vi "Create user events.vi"(8 "error in (no error)":errorcluster) -> (0 "error out":errorcluster, 3 "User events":T1)   [LabVIEW 2020, in "NI DAQ.lvlib"]
uses:
  NI DAQ.lvlib
  Task list.ctl
  Continuous aquisition params.ctl
  Controls/Acuisition type --typedef.ctl
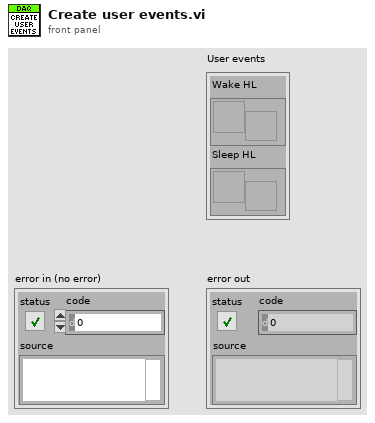
[diagram p1: front panel]
types:
  T1 = cluster{"Wake HL":refnum<user-event>, "Sleep HL":refnum<user-event>}
  T2 = typedef "NI DAQ.lvlib/Continuous aquisition params.ctl" = cluster{"Module ID":i32, "Task list":T3, "Timeout":i32, "Data in":variant, "DAQmx Task":refnum<k21>, "N samples":i32, "Acq type":T4}
  T3 = typedef "NI DAQ.lvlib/Task list.ctl" = enum16{"All", "DO task", "DI task", "AO task", "AI task", "CI task", "CO task", "TC task"}
  T4 = typedef "NI DAQ.lvlib/Acuisition type --typedef.ctl" = enum16{"Single", "Average", "Multiple"}
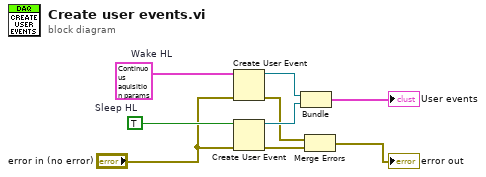
[diagram p0: block diagram]
diagram:
  w6 = TRUE  # Sleep HL
  w5 = T2 {"Module ID"=0, "Task list"=enum."All", "Timeout"=0, "Data in"=variant, "DAQmx Task"="", "N samples"=0, "Acq type"=enum."Single"}  # Wake HL
  n1 = Create User Event(user event datatype=w5, error in="error in (no error)") -> (user event=w7:refnum<user-event>, error out=w3:errorcluster)
  n2 = Create User Event(user event datatype=w6, error in="error in (no error)") -> (user event=w8:refnum<user-event>, error out=w2:errorcluster)
  n3 = Bundle("Wake HL"=w7, "Sleep HL"=w8) -> (→"User events":T1)  [unwired: 1 in]
  n4 = Merge Errors(w3, w2) -> (→"error out":errorcluster)
